vi "Calibration.vi"() -> ()   [LabVIEW 2018]
uses:
  <vilib>/Analysis/6fits.llb/Curve Fitting Criteria.ctl
  <vilib>/Analysis/NI_AALPro.lvlib
panel:
  out "residue":dbl
  out "intercept":dbl format="%.3f"
  out "slope":dbl format="%.3f"
  out "Multiple Plots":cluster{dbl[], "Best Linear Fit":dbl[]}[](graph)
  in  "Calibrate Button":bool
  in  "Data":dbl[][](array[numeric])
  in  "Stop":bool
  in  "Insert":bool
  in  "Reference":dbl
  in  "Raw":dbl
  # "RAW DATA (A)"
  # "REF READING (PSI)"
  # "CAL READING (PSI)"
  # "X +"
  # "Notes:\n1. Raw data needs to be averaged on cRIO before send to UI"
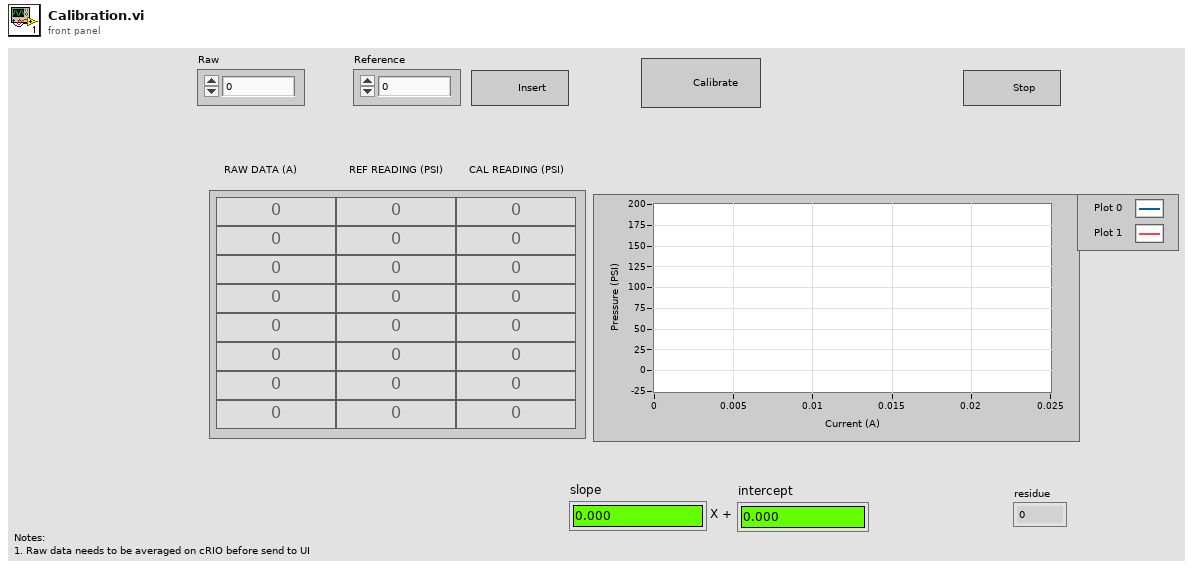
[diagram p1: front panel]
types:
  T1 = typedef "NI_AALPro.lvlib/Curve Fitting Criteria.ctl" = u16
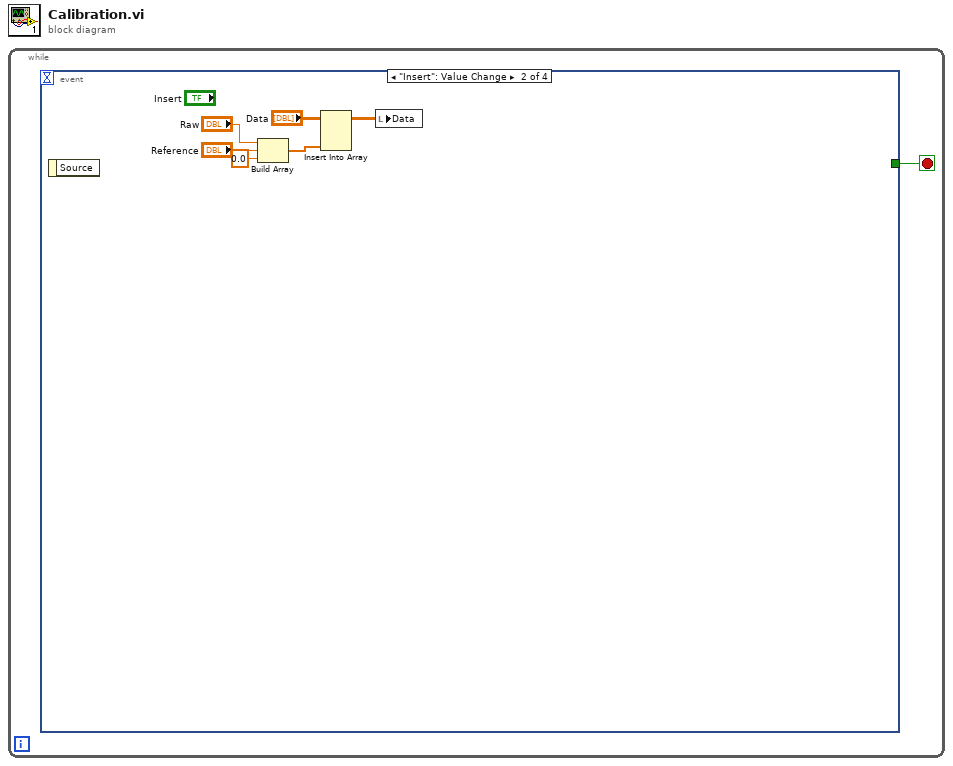
[diagram p0: block diagram]
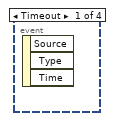
[diagram p2: hidden frame]
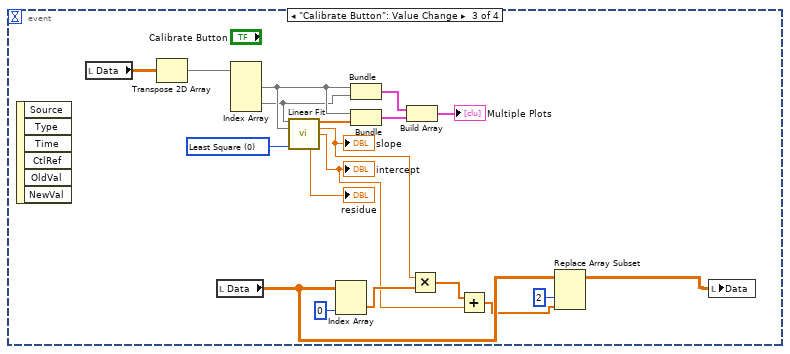
[diagram p3: hidden frame]
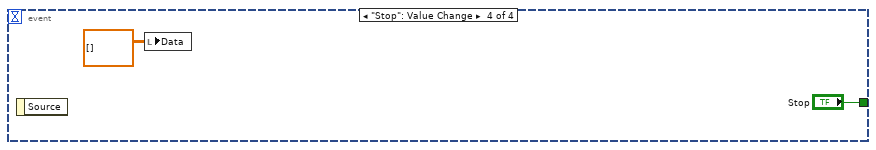
[diagram p4: hidden frame]
diagram:
  n1 = while {
    stop <- w1 stop-if-true
    n2 = event shown="[1] \"Insert\": Value Change" {
      selector: _ -> [_ _ _ _]
      dyn-events: _ -> [_ _ _ _]
      timeout: _ -> [_ _ _ _]
      tunnel: [_ _ _ "Stop"] -> w1
      event Timeout {
        n3 = event-data() -> ()  [unwired: 1 in, 3 out]
      }
      event "Insert": Value Change {
        n4 = event-data() -> ()  [unwired: 1 in, 1 out]
        n5 = Build Array("Raw", "Reference", 0.0 ("element")) -> (w4:dbl[])
        n6 = Insert Into Array(array="Data", new element=w4) -> (w3:dbl[][])  [unwired: 2 in]
        n7 = local write "Data"(w3) -> ()
      }
      event "Calibrate Button": Value Change {
        w26 = T1 0 items=["Least Square", "Least Absolute Residual", "Bisquare"] ("method")
        n8 = event-data() -> ()  [unwired: 1 in, 6 out]
        n9 = local read "Data"() -> (w24:dbl[][])
        n10 = Transpose 2D Array(2D array=w24) -> (transposed array=w25:dbl[][])
        n11 = local read "Data"() -> (w11:dbl[][])
        n12 = Index Array(array=w25) -> (element #1=w19:dbl[], element #2=w18:dbl[])  [unwired: 4 in]
        n13 = call <vilib>:"Linear Fit.vi"("Y"=w18, "X"=w19, "method"=w26) -> ("Best Linear Fit"=w21:dbl[], "slope"=w14:dbl, "intercept"=w12:dbl, "residue"=→"residue":dbl)  [unwired: 8 in, 1 out]
        "slope" <- w14
        "intercept" <- w12
        n14 = Index Array(array=w11, index (col)=0 ("disabled index (col)")) -> (element=w15:dbl[])  [unwired: 1 in]
        n15 = Bundle(w19, w18) -> (w22:cluster{dbl[], dbl[]})  [unwired: 1 in]
        n16 = Bundle(w19, "Best Linear Fit"=w21) -> (w20:cluster{dbl[], "Best Linear Fit":dbl[]})  [unwired: 1 in]
        n17 = Build Array(w22, w20) -> (→"Multiple Plots":cluster{dbl[], "Best Linear Fit":dbl[]}[])
        n18 = Multiply(x=w14, y=w15) -> (x*y=w13:dbl[])
        n19 = Add(x=w13, y=w12) -> (x+y=w9:dbl[])
        n20 = Replace Array Subset(array=w11, new element=w9, index (col)=2 ("disabled index (col)")) -> (w8:dbl[][])  [unwired: 1 in]
        n21 = local write "Data"(w8) -> ()
      }
      event "Stop": Value Change {
        n22 = event-data() -> ()  [unwired: 1 in, 1 out]
        n23 = local write "Data"(dbl[][] [] ("Data")) -> ()
      }
    }
  }
